vi "Configure TV Trigger Source [TV] Core.vi"(0 "CS++Scope":refnum<class "CS++Scope.lvclass">, 1 "trigger source (\"CHANNEL1\")":string(combo)="CHANNEL1", 2 "tv event (Field 1)":i32(ring)=1 items=["Field 1"=1, "Field 2"=2, "Any Field"=3, "Any Line"=4, "Line Number"=5], 3 "tv trigger polarity (Positive)":i32(ring)=1 items=["Positive"=1, "Negative"=2], 4 "tv signal format (NTSC)":i32(ring)=1 items=["NTSC"=1, "PAL"=2, "SECAM"=3], 5 "error in (no error)":errorcluster) -> (14 "CS++Scope out":refnum<class "CS++Scope.lvclass">, 19 "error out":errorcluster)   [LabVIEW 2013, in "CS++Scope.lvlib" / "CS++Scope.lvclass"]
doc: "This VI configures the oscilloscope for TV triggering. It configures the TV signal format, the event and the signal polarity."
uses:
  CS++Scope.lvclass
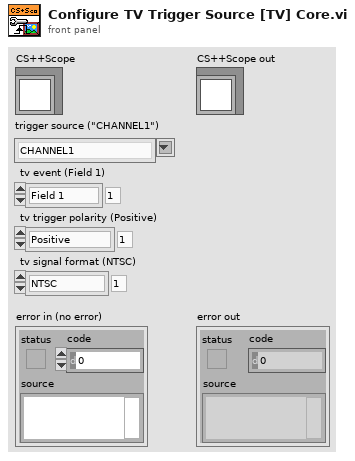
[diagram p1: front panel]
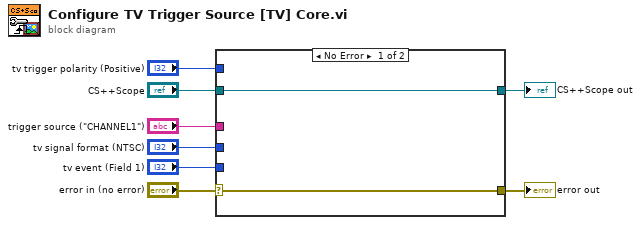
[diagram p0: block diagram]
diagram:
  n1 = case shown="No Error" "error in (no error)" {
    selector: "error in (no error)" -> [w9 w12]
    tunnel: [w9 w12] -> w7
    tunnel: [w10 w11] -> w2
    tunnel: "CS++Scope" -> [w10 w11]
    tunnel: "trigger source (\"CHANNEL1\")" -> [_ _]
    tunnel: "tv signal format (NTSC)" -> [_ _]
    tunnel: "tv event (Field 1)" -> [_ _]
    tunnel: "tv trigger polarity (Positive)" -> [_ _]
    frame No Error {
    }
    frame Error {
    }
  }
  "error out" <- w7
  "CS++Scope out" <- w2
